vi "UIMessage.vi"(4 "?":refnum<vi>, 5 "Event Data":cluster{"uiMsg":refnum<k7>, "cancel":bool}, 6 "Control Ref":refnum<k7>, 7 "Event Common Data":T1) -> (1 "Event Data Out":cluster{"cancel":bool})   [LabVIEW 2018]
uses:
  <vilib>/Utility/miscctls.llb/LVRowAndColumnUnsignedTypeDef.ctl
  <vilib>/Utility/miscctls.llb/LVRowAndColumnTypeDef.ctl
panel:
  in  "error in (no error)":errorcluster
  out "reference out":refnum<vi>
  out "error out":errorcluster
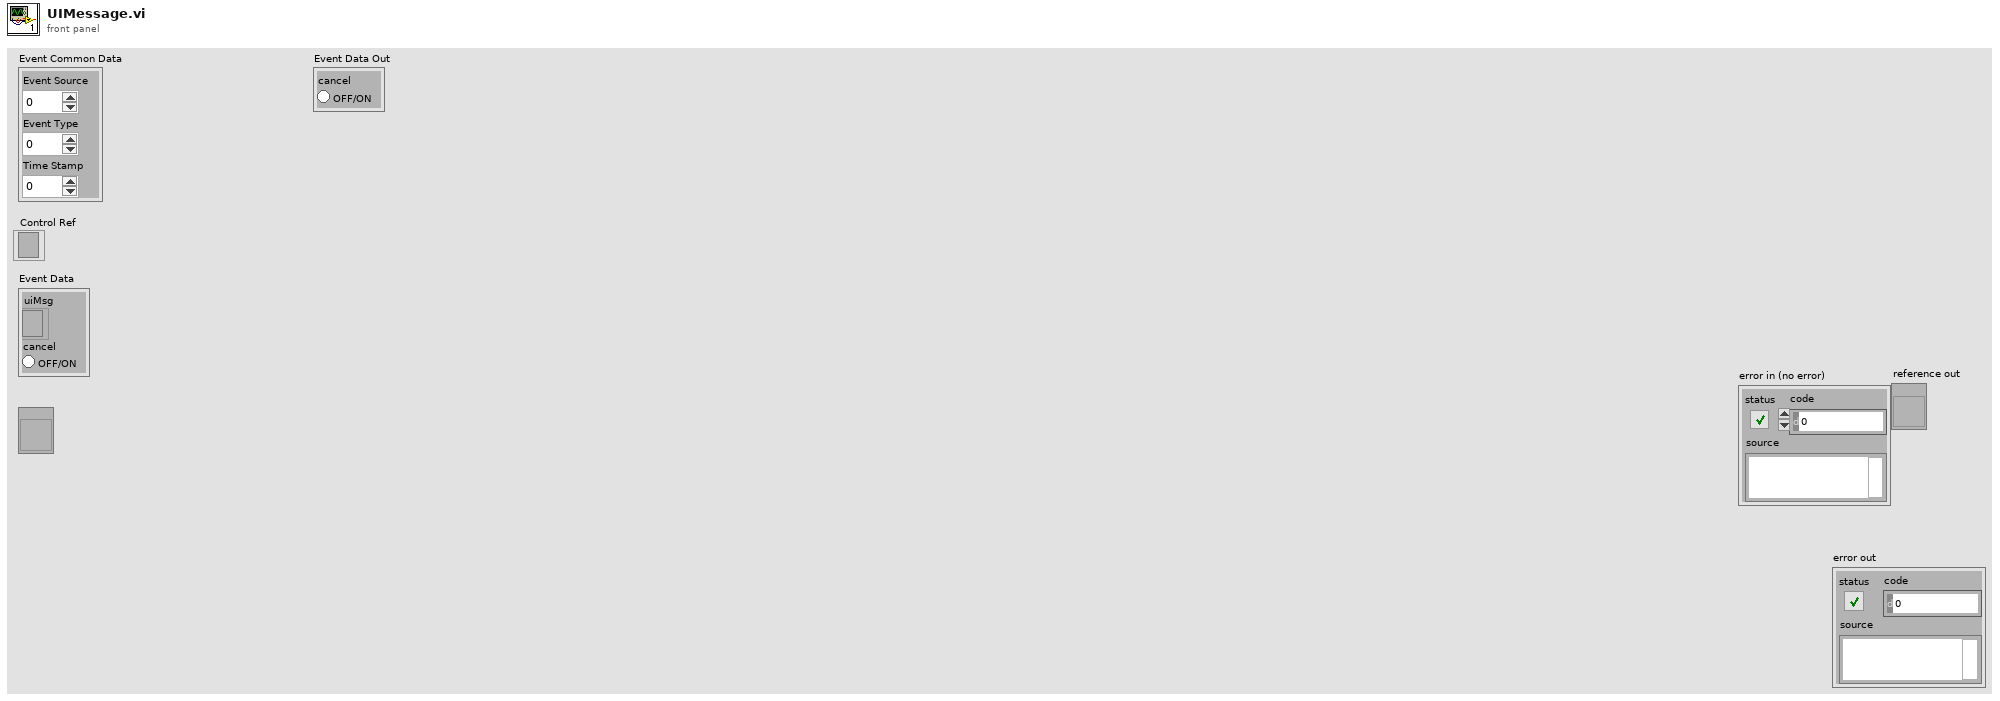
[diagram p1: front panel]
types:
  T1 = cluster{"Event Source":i32, "Event Type":u32, "Time Stamp":u32}
  T2 = typedef "LVRowAndColumnUnsignedTypeDef.ctl" = cluster{"Row":u32, "Column":u32}
  T3 = typedef "LVRowAndColumnTypeDef.ctl" = cluster{"Row":i32, "Column":i32}
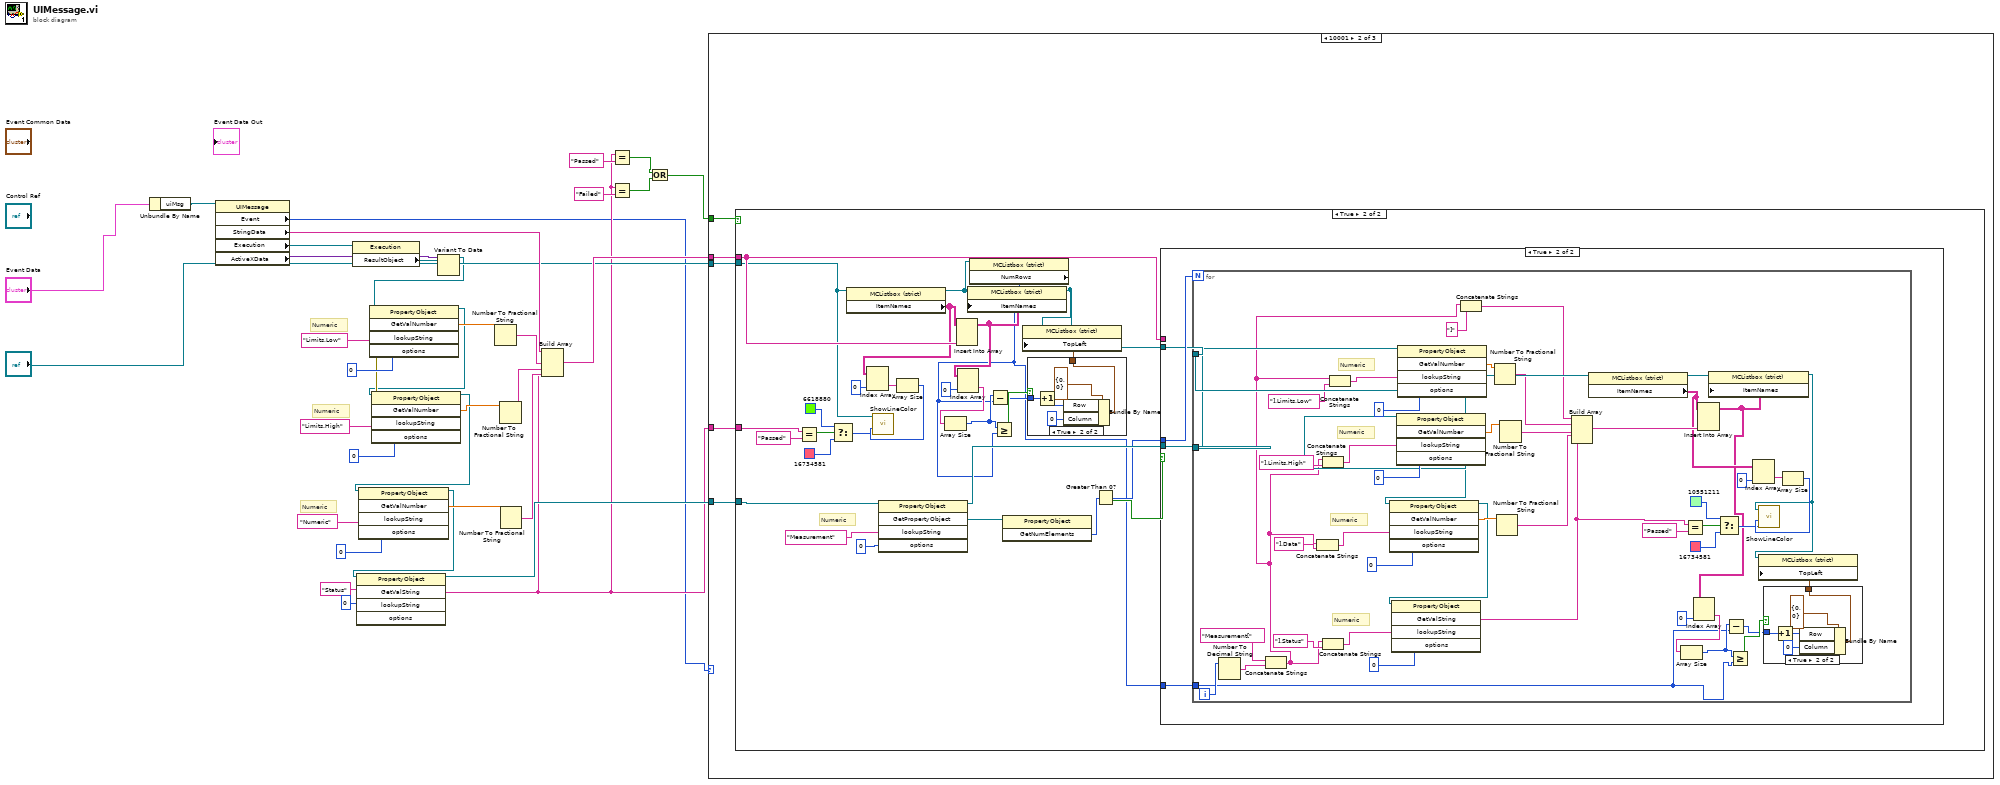
[diagram p0: block diagram]
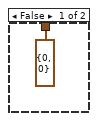
[diagram p4: hidden frame]
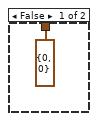
[diagram p6: hidden frame]
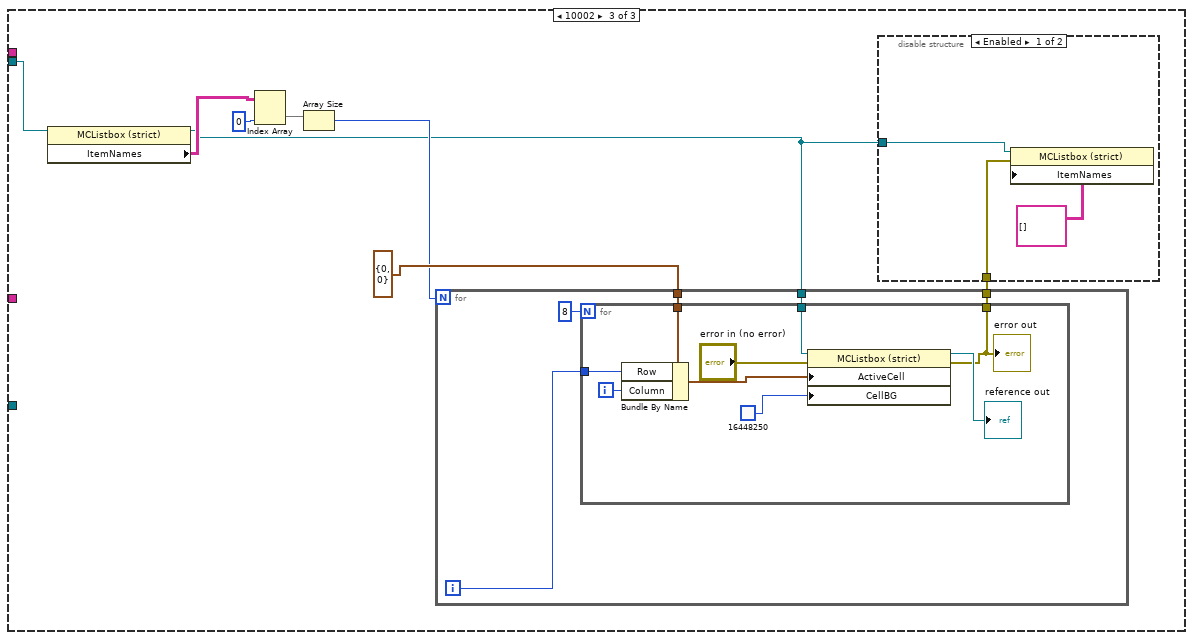
[diagram p7: hidden frame]
diagram:
  # "Numeric"
  # "Numeric"
  # "Numeric"
  n1 = Unbundle By Name("Event Data") -> ("uiMsg"=w35:refnum<k7>)
  n2 = property class="UIMessage"(reference=w35) -> ("Event"=w2:i32, "StringData"=w27:string, "Execution"=w31:refnum<k7>, "ActiveXData"=w34:variant)  [unwired: 1 in, 2 out]
  n3 = property class="Execution"(reference=w31) -> ("ResultObject"=w30:refnum<k7>)  [unwired: 1 in, 2 out]
  n4 = Variant To Data(type=w30, Variant=w34) -> (data=w12:refnum<k7>)  [unwired: 1 in, 1 out]
  n5 = invoke class="PropertyObject" method="GetValNumber"(reference=w12, "lookupString"="Limits.Low", "options"=0) -> (reference out=w11:refnum<k7>, error out=w16:errorcluster, "GetValNumber"=w21:dbl)  [unwired: 2 in, 2 out]
  n6 = invoke class="PropertyObject" method="GetValNumber"(reference=w11, error in=w16, "lookupString"="Limits.High", "options"=0) -> (reference out=w10:refnum<k7>, "GetValNumber"=w19:dbl)  [unwired: 1 in, 3 out]
  n7 = invoke class="PropertyObject" method="GetValNumber"(reference=w10, "lookupString"="Numeric", "options"=0) -> (reference out=w9:refnum<k7>, "GetValNumber"=w25:dbl)  [unwired: 2 in, 3 out]
  n8 = invoke class="PropertyObject" method="GetValString"(reference=w9, "lookupString"="Status", "options"=0) -> (reference out=w8:refnum<k7>, "GetValString"=w3:string)  [unwired: 2 in, 3 out]
  n9 = Number To Fractional String(number=w21) -> (F-format string=w20:string)  [unwired: 3 in]
  n10 = Number To Fractional String(number=w19) -> (F-format string=w13:string)  [unwired: 3 in]
  n11 = Number To Fractional String(number=w25) -> (F-format string=w24:string)  [unwired: 3 in]
  n12 = Build Array(w27, w20, w13, w24, w3) -> (w15:string[])
  n13 = Equal?(x=w3, y="Passed") -> (x = y?=w5:bool)
  n14 = Equal?(x=w3, y="Failed") -> (x = y?=w4:bool)
  n15 = Or(x=w5, y=w4) -> (x .or. y?=w1:bool)
  n16 = case shown="10001" w2 {
    tunnel: w15 -> [_ w40 _]
    tunnel: "?" -> [_ w39 w139]
    tunnel: w1 -> [_ w38 _]
    tunnel: w8 -> [_ w37 _]
    tunnel: w3 -> [_ w36 _]
    frame 0, Default {
    }
    frame 10001 {
      n17 = case shown="True" w38 {
        tunnel: w40 -> [_ w68]
        tunnel: w39 -> [_ w61]
        tunnel: w37 -> [_ w64]
        tunnel: w36 -> [_ w52]
        frame False {
        }
        frame True {
          # "Numeric"
          n18 = Equal?(x=w52, y="Passed") -> (x = y?=w55:bool)
          n19 = Select(t=u32 6618880, s=w55, f=u32 16734581) -> (s? t:f=w51:u32)
          n20 = property on="Property Node" class="MCListbox (strict)"(reference=w61) -> (reference out=w42:refnum<vi>, "ItemNames"=w60:string[][])  [unwired: 1 in, 1 out]
          n21 = Index Array(array=w60, index (col)=0 ("disabled index (col)")) -> (element=w58:string[])  [unwired: 1 in]
          n22 = invoke class="PropertyObject" method="GetPropertyObject"(reference=w64, "lookupString"="Measurement", "options"=0) -> (reference out=w63:refnum<k7>, "GetPropertyObject"=w67:refnum<k7>)  [unwired: 2 in, 3 out]
          n23 = Array Size(array=w58) -> (size(s)=w57:i32)
          n24 = call "ShowLineColor.vi"("ColorIn"=w51, "TestingIndex"=w57, "MulticolumnListbox in"=w61) -> ()  [unwired: 9 in]
          n25 = Insert Into Array(array=w60, new element=w68) -> (w49:string[][])  [unwired: 2 in]
          n26 = Index Array(array=w49, index (col)=0 ("disabled index (col)")) -> (element=w47:string[])  [unwired: 1 in]
          n27 = Array Size(array=w47) -> (size(s)=w45:i32)
          n28 = property on="Property Node" class="MCListbox (strict)"(reference=w42, "ItemNames"=w49) -> (reference out=w50:refnum<vi>)  [unwired: 1 in, 1 out]
          n29 = property on="Property Node" class="MCListbox (strict)"(reference=w42) -> ("NumRows"=w41:u32)  [unwired: 1 in, 2 out]
          n30 = Subtract(x=w45, y=w41) -> (x-y=w43:u32)
          n31 = Greater Or Equal?(x=w45, y=w41) -> (x >= y?=w46:bool)
          n32 = invoke class="PropertyObject" method="GetNumElements"(reference=w67) -> ("GetNumElements"=w62:i32)  [unwired: 2 in, 2 out]
          n33 = case shown="True" w46 {
            tunnel: [T2 {"Row"=0, "Column"=0} ("Top Left Visible Cell") w73] -> w44
            tunnel: w43 -> [_ w72]
            frame False {
            }
            frame True {
              n34 = Increment(x=w72) -> (x+1=w71:u32)
              n35 = Bundle By Name(cluster=T2 {"Row"=0, "Column"=0} ("Top Left Visible Cell"), "Row"=w71, "Column"=u32 0) -> (w73:T2)
            }
          }
          n36 = property class="MCListbox (strict)"(reference=w50, "TopLeft"=w44) -> ()  [unwired: 1 in, 2 out]
          n37 = Greater Than 0?(x=w62) -> (x > 0?=w69:bool)
          n38 = case shown="True" w69 {
            tunnel: w62 -> [_ w79]
            tunnel: w63 -> [_ w78]
            tunnel: w68 -> [_ _]
            tunnel: w50 -> [_ w77]
            tunnel: w41 -> [_ w76]
            frame False {
            }
            frame True {
              n39 = for {
                N: w79 -> [_]
                tunnel: w78 -> [w116]
                tunnel: w77 -> [w129]
                tunnel: w76 -> [w80]
                i -> [w113]
                # "Numeric"
                # "Numeric"
                # "Numeric"
                # "Numeric"
                n40 = Number To Decimal String(number=w113) -> (decimal integer string=w112:string)  [unwired: 1 in]
                n41 = Concatenate Strings("Measurement[" ("string"), w112) -> (w101:string)
                n42 = Concatenate Strings(w101, "].Data" ("lookupString")) -> (w105:string)
                n43 = Concatenate Strings(w101, "].Limits.High" ("lookupString")) -> (w107:string)
                n44 = Concatenate Strings(w101, "].Status" ("lookupString")) -> (w103:string)
                n45 = Concatenate Strings(w101, "].Limits.Low" ("lookupString")) -> (w109:string)
                n46 = invoke class="PropertyObject" method="GetValNumber"(reference=w116, "lookupString"=w109, "options"=0) -> (reference out=w124:refnum<k7>, "GetValNumber"=w126:dbl)  [unwired: 2 in, 3 out]
                n47 = invoke class="PropertyObject" method="GetValNumber"(reference=w124, "lookupString"=w107, "options"=0) -> (reference out=w117:refnum<k7>, "GetValNumber"=w122:dbl)  [unwired: 2 in, 3 out]
                n48 = invoke class="PropertyObject" method="GetValNumber"(reference=w117, "lookupString"=w105, "options"=0) -> (reference out=w114:refnum<k7>, "GetValNumber"=w120:dbl)  [unwired: 2 in, 3 out]
                n49 = invoke class="PropertyObject" method="GetValString"(reference=w114, "lookupString"=w103, "options"=0) -> ("GetValString"=w90:string)  [unwired: 2 in, 4 out]
                n50 = Concatenate Strings(w101, "]" ("string")) -> (w100:string)
                n51 = Number To Fractional String(number=w126) -> (F-format string=w123:string)  [unwired: 3 in]
                n52 = Number To Fractional String(number=w120) -> (F-format string=w118:string)  [unwired: 3 in]
                n53 = Number To Fractional String(number=w122) -> (F-format string=w121:string)  [unwired: 3 in]
                n54 = Build Array(w100, w123, w121, w118, w90) -> (w128:string[])
                n55 = property on="Property Node" class="MCListbox (strict)"(reference=w129) -> (reference out=w102:refnum<vi>, "ItemNames"=w91:string[][])  [unwired: 1 in, 1 out]
                n56 = Equal?(x=w90, y="Passed") -> (x = y?=w96:bool)
                n57 = Insert Into Array(array=w91, new element=w128) -> (w84:string[][])  [unwired: 2 in]
                n58 = Index Array(array=w84, index (col)=0 ("disabled index (col)")) -> (element=w86:string[])  [unwired: 1 in]
                n59 = Array Size(array=w86) -> (size(s)=w87:i32)
                n60 = property on="Property Node" class="MCListbox (strict)"(reference=w102, "ItemNames"=w84) -> (reference out=w82:refnum<vi>)  [unwired: 1 in, 1 out]
                n61 = Select(t=u32 10551211, s=w96, f=u32 16734581) -> (s? t:f=w89:u32)
                n62 = Subtract(x=w87, y=w80) -> (x-y=w81:u32)
                n63 = Greater Or Equal?(x=w87, y=w80) -> (x >= y?=w83:bool)
                n64 = Index Array(array=w91, index (col)=0 ("disabled index (col)")) -> (element=w93:string[])  [unwired: 1 in]
                n65 = case shown="True" w83 {
                  tunnel: [T2 {"Row"=0, "Column"=0} ("Top Left Visible Cell") w133] -> w88
                  tunnel: w81 -> [_ w132]
                  frame False {
                  }
                  frame True {
                    n66 = Increment(x=w132) -> (x+1=w131:u32)
                    n67 = Bundle By Name(cluster=T2 {"Row"=0, "Column"=0} ("Top Left Visible Cell"), "Row"=w131, "Column"=u32 0) -> (w133:T2)
                  }
                }
                n68 = property class="MCListbox (strict)"(reference=w82, "TopLeft"=w88) -> ()  [unwired: 1 in, 2 out]
                n69 = Array Size(array=w93) -> (size(s)=w94:i32)
                n70 = call "ShowLineColor.vi"("ColorIn"=w89, "TestingIndex"=w94, "MulticolumnListbox in"=w82) -> ()  [unwired: 9 in]
              }
            }
          }
        }
      }
    }
    frame 10002 {
      n71 = property class="MCListbox (strict)"(reference=w139) -> (reference out=w137:refnum<vi>, "ItemNames"=w138:string[][])  [unwired: 1 in, 1 out]
      n72 = Index Array(array=w138, index (col)=0 ("disabled index (col)")) -> (element=w141:string[])  [unwired: 1 in]
      n73 = Array Size(array=w141) -> (size(s)=w140:i32)
      n74 = for {
        N: w140 -> [_]
        tunnel: T3 {"Row"=0, "Column"=0} ("Active Cell:Active Cell") -> [w151]
        tunnel: [w150] -> w136
        tunnel: w137 -> [w147]
        i -> [w148]
        n75 = for {
          N: 8 -> [_]
          tunnel: w148 -> [w159]
          tunnel: w151 -> [w158]
          tunnel: [w153] -> w150
          tunnel: w147 -> [w152]
          i -> [w157]
          n76 = Bundle By Name(cluster=w158, "Row"=w159, "Column"=w157) -> (w160:T3)
          n77 = property on="Property Node" class="MCListbox (strict)"(reference=w152, error in="error in (no error)", "ActiveCell"=w160, "CellBG"=u32 16448250) -> (reference out=→"reference out":refnum<vi>, error out=w153:errorcluster)
          "error out" <- w153
        }
      }
      n78 = disable-structure shown="Enabled" {
        disable-tunnel: w137 -> [w146 _]
        disable-tunnel: w136 -> [w145 _]
        frame Enabled {
          n79 = property class="MCListbox (strict)"(reference=w146, error in=w145, "ItemNames"=string[][] [] ("Item Names")) -> ()  [unwired: 2 out]
        }
        frame Disabled {
        }
      }
    }
  }
